vi "LAKESHORE_10_01_2023_R_VS_T_DEMO_2.vi"() -> ()   [LabVIEW 2020]
panel:
  out "Temperature":dbl
  in  "Average Number of readings \nper iterations":i32
  in  "Stop Button":bool
  in  "Save data":bool
  in  "File_name":path=path "saved_data"
  out "Resistance":dbl
  in  "Channel 2":T1(ring)
  out "XY Graph":cluster{"X":dbl[], "Y":dbl[]}[](graph)
  in  "VISA resource name 2":refnum<visa-resource-name>
  # "LAKE SHORE 372"
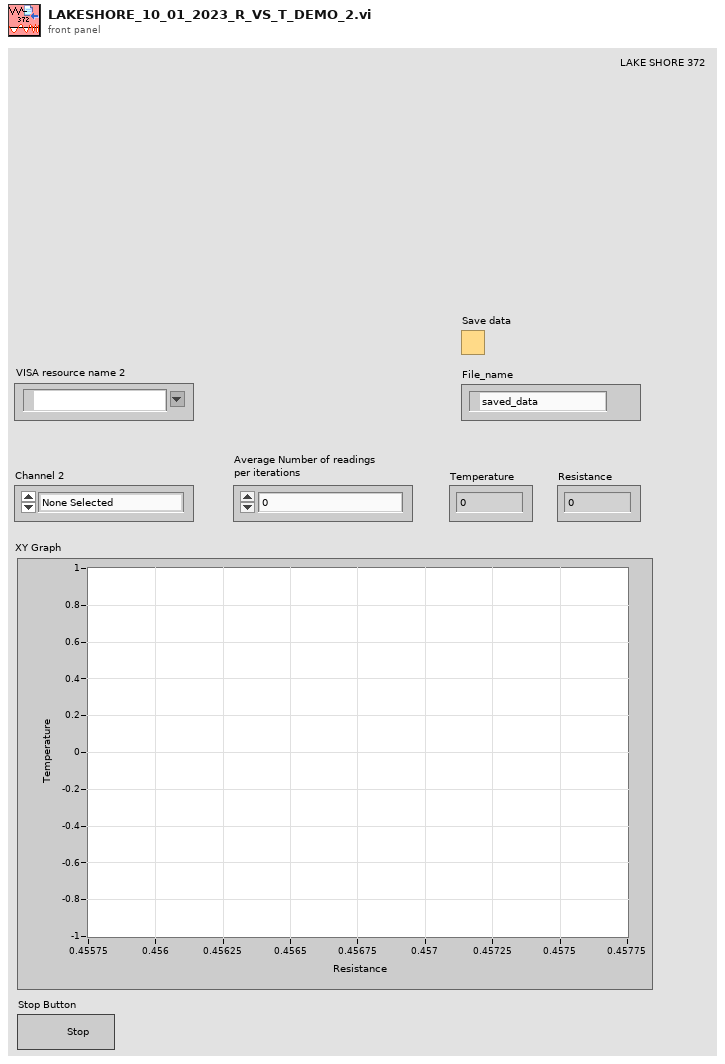
[diagram p1: front panel]
types:
  T1 = enum16{"None Selected", "1", "2", "3", "4", "5", "6", "7", "8", "9", "10", "11", "12", "13", "14", "15", "16"}
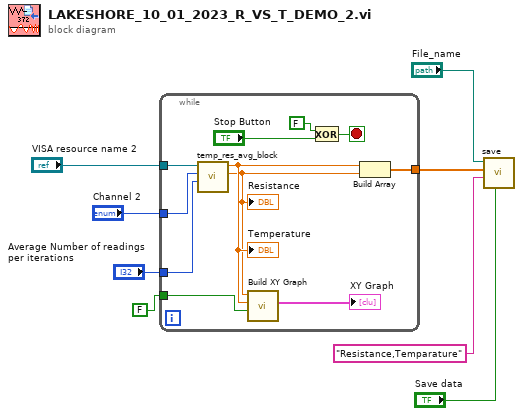
[diagram p0: block diagram]
diagram:
  n1 = while {
    tunnel: "VISA resource name 2" -> [w13]
    tunnel: FALSE ("Reset") -> [w18]
    tunnel: "Channel 2" -> [w12]
    tunnel: [w17] -> w1
    tunnel: "Average Number of readings \nper iterations" -> [w11]
    stop <- w14 stop-if-true
    n2 = call "temp_res_avg_block.vi"("Avg"=w11, "Channel in"=w12, "VISA Refnum in"=w13) -> ("Numeric"=w9:dbl, "Numeric 2"=w10:dbl)  [unwired: 7 in]
    "Resistance" <- w9
    "Temperature" <- w10
    n3 = call "Build XY Graph"("Reset"=w18, "Y Input"=w10, "X Input"=w9) -> ("XY Graph"=→"XY Graph":cluster{"X":dbl[], "Y":dbl[]}[])  [unwired: 7 in, 1 out]
    n4 = Exclusive Or(1:"Stop Button", 2:FALSE) -> (0:w14:bool)
    n5 = Build Array(w10, w9) -> (w17:dbl[])
  }
  n6 = call "save.vi"("Save data"="Save data", "String"="Resistance,Temparature", "Array"=w1, "File_name"="File_name") -> ()  [unwired: 8 in]
